vi "write (CryoCon_no open).vi"(2 "error in (no error)":errorcluster, 3 "write buffer":string) -> (0 "error out":errorcluster, 1 "VISA resource name out":refnum<visa-resource-name>)   [LabVIEW 2011]
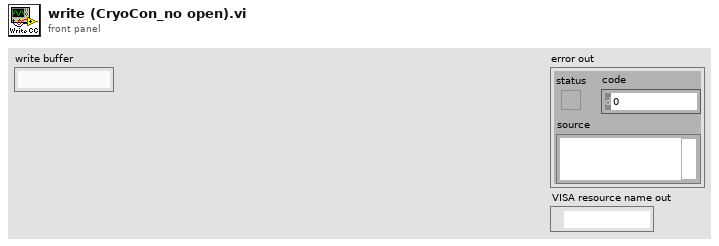
[diagram p1: front panel]
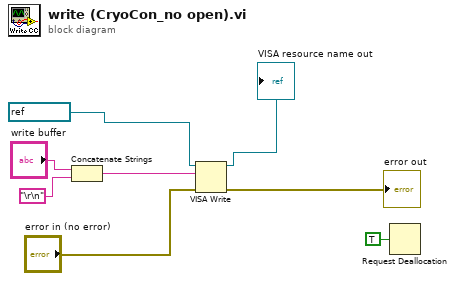
[diagram p0: block diagram]
diagram:
  n1 = Concatenate Strings("write buffer", "\r\n") -> (w5:string)
  n2 = VISA Write(VISA resource name=refnum<visa-resource-name> "COM3", write buffer=w5, error in (no error)="error in (no error)") -> (VISA resource name out=→"VISA resource name out":refnum<visa-resource-name>, error out=→"error out":errorcluster)  [unwired: 1 out]
  n3 = Request Deallocation(TRUE ("flag")) -> ()
